vi "PID Set Points.vi"() -> ()   [LabVIEW 2011]
panel:
  out "Hood Voltage":dbl
  out "Indexer Set Speed":dbl
  out "ShooterSet Speed":dbl
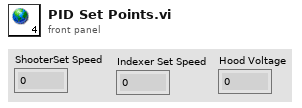
[diagram p1: front panel]
diagram:
